vi "Get Server State UE.vi"(11 "Template Server in":refnum<class "ctet_mux.lvclass">) -> (2 "Server Internal State UE":refnum<user-event>, 3 "Template Server out":refnum<class "ctet_mux.lvclass">)   [LabVIEW 2019, in "ctet_mux.lvlib" / "ctet_mux.lvclass"]
uses:
  ctet_mux.lvclass
  typeDefs/Server State Data.ctl
  ctet_mux.lvclass/ctet_mux.ctl
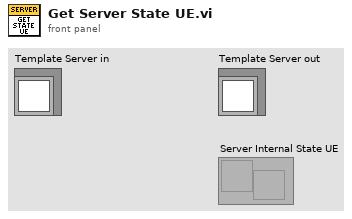
[diagram p1: front panel]
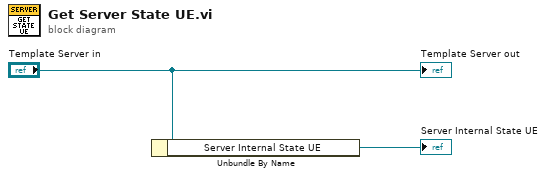
[diagram p0: block diagram]
diagram:
  n1 = Unbundle By Name("Template Server in") -> ("Server Internal State UE"=→"Server Internal State UE":refnum<user-event>)
  "Template Server out" <- "Template Server in"
